vi "RemoveAllWorksheetsExcept.vi"(8 "error in (no error)":errorcluster, 9 "Worksheet Name":string, 11 "ExcelFile in":refnum<class "PortableExcelFileManipulationOXML.lvclass">) -> (0 "error out":errorcluster, 3 "ExcelFile out":refnum<class "PortableExcelFileManipulationOXML.lvclass">)   [LabVIEW 2019, in "PortableExcelFileManipulationOXML.lvclass"]
doc: "Adds a worksheet to the This excel File by name."
uses:
  PortableExcelFileManipulationOXML.lvclass
  PortableExcelFileManipulationOXML.lvclass/PortableExcelFileManipulationOXML.ctl
  H:/LV projects/ExpressionEvaluator/Excel/ExcelManipulation.dll
  ExcelManipulation.dll
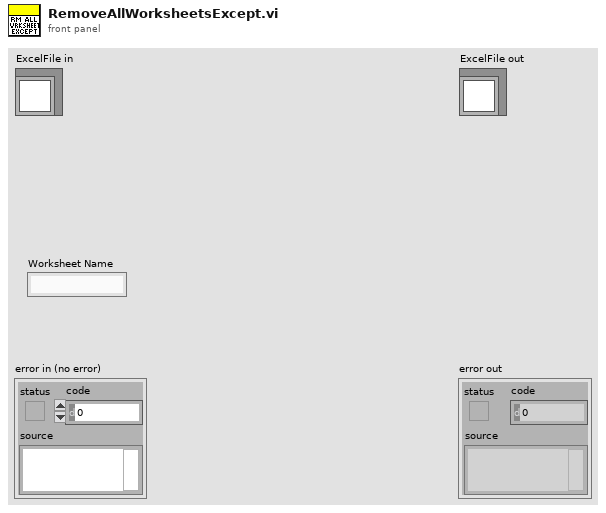
[diagram p1: front panel]
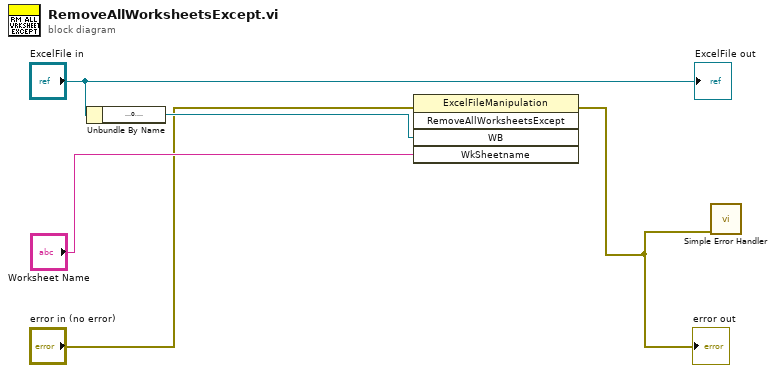
[diagram p0: block diagram]
diagram:
  n1 = Unbundle By Name("ExcelFile in") -> ("ExcelOpen"=w4:refnum<k24>)
  n2 = invoke class="ExcelFileManipulation" method="RemoveAllWorksheetsExcept"(error in="error in (no error)", "WB"=w4, "WkSheetname"="Worksheet Name") -> (error out=w1:errorcluster)  [unwired: 2 in, 4 out]
  "error out" <- w1
  n3 = call <vilib>:"Simple Error Handler.vi"("error in (no error)"=w1) -> ()  [unwired: 4 in, 5 out]
  "ExcelFile out" <- "ExcelFile in"
